vi "Write Section.vi"(8 "error in":errorcluster, 10 "Section":string, 11 "Text Device Session in":refnum<class "Text Device Session.lvclass">) -> (0 "error out":errorcluster, 3 "Text Device Session out":refnum<class "Text Device Session.lvclass">)   [LabVIEW 2014, in "Text Device Session.lvclass"]
uses:
  Text Device Session.lvclass
  Text Device Session.lvclass/Text Device Session.ctl
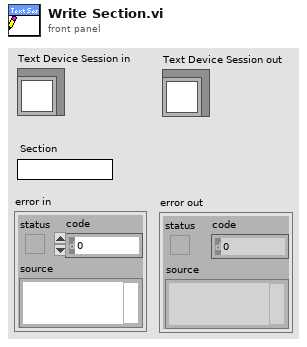
[diagram p1: front panel]
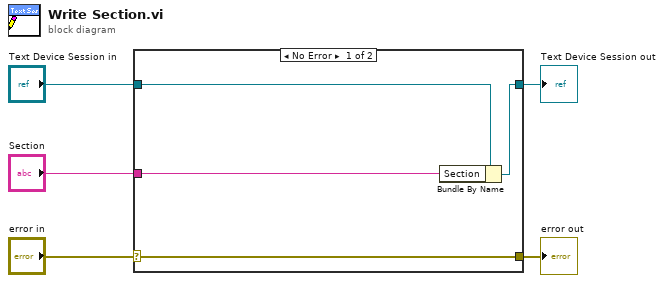
[diagram p0: block diagram]
diagram:
  n1 = case shown="No Error" "error in" {
    selector: "error in" -> [w9 w10]
    tunnel: [w9 w10] -> w4
    tunnel: [w7 w11] -> w2
    tunnel: "Text Device Session in" -> [w8 w11]
    tunnel: "Section" -> [w6 _]
    frame No Error {
      n2 = Bundle By Name(cluster=w8, "Section"=w6) -> (w7:refnum<class "Text Device Session.lvclass">)
    }
    frame Error {
    }
  }
  "error out" <- w4
  "Text Device Session out" <- w2
